vi "uncertainty_array.vi"(6 "unc_2":dbl[](array[numeric]), 7 "unc_1":dbl[](array[numeric])) -> (0 "max_unc":dbl, 2 "Array_unc":dbl[](array[numeric]))   [LabVIEW 2021]
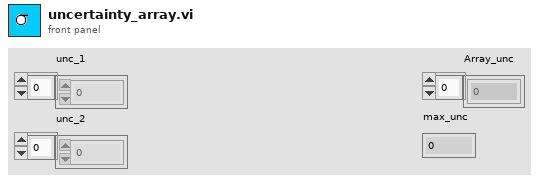
[diagram p1: front panel]
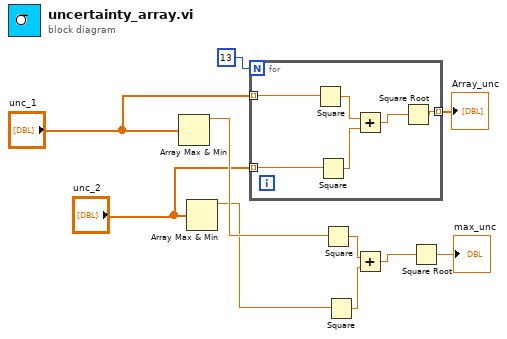
[diagram p0: block diagram]
diagram:
  n1 = Array Max & Min(array="unc_1") -> (max value=w6:dbl)  [unwired: 3 out]
  n2 = Array Max & Min(array="unc_2") -> (max value=w5:dbl)  [unwired: 3 out]
  n3 = for {
    N: 13 -> [_]
    tunnel: [w13] -> w2 mode=indexing
    tunnel: "unc_1" -> [w12] mode=indexing
    tunnel: "unc_2" -> [w11] mode=indexing
    n4 = Square(x=w12) -> (x^2=w16:dbl)
    n5 = Square(x=w11) -> (x^2=w15:dbl)
    n6 = Add(x=w16, y=w15) -> (x+y=w14:dbl)
    n7 = Square Root(x=w14) -> (sqrt(x)=w13:dbl)
  }
  "Array_unc" <- w2
  n8 = Square(x=w6) -> (x^2=w7:dbl)
  n9 = Square(x=w5) -> (x^2=w8:dbl)
  n10 = Add(x=w7, y=w8) -> (x+y=w9:dbl)
  n11 = Square Root(x=w9) -> (sqrt(x)=→"max_unc":dbl)
